vi "ShiftReg.vi"() -> ()   [LabVIEW 2012]
uses:
  <vilib>/Waveform/DTblOps.llb/DTbl Boolean Array to Digital.vi
panel:
  in  "D":bool
  out "Digital Waveform Graph":digitaldata(graph)
  in  "millisecond multiple":u32
  out "Q4":bool
  out "Q3":bool
  out "Clk":bool
  out "Q2":bool
  in  "Slices":u32
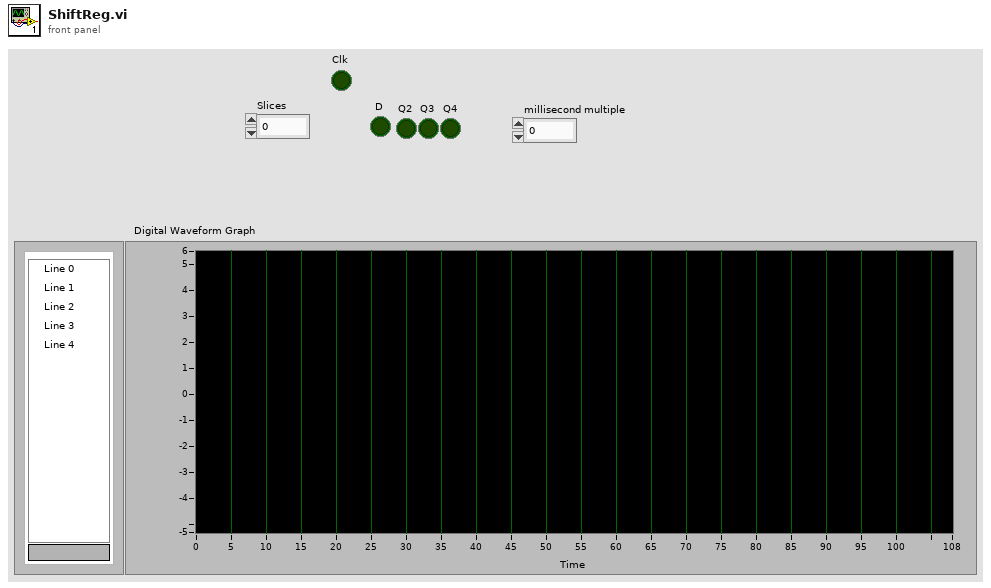
[diagram p1: front panel]
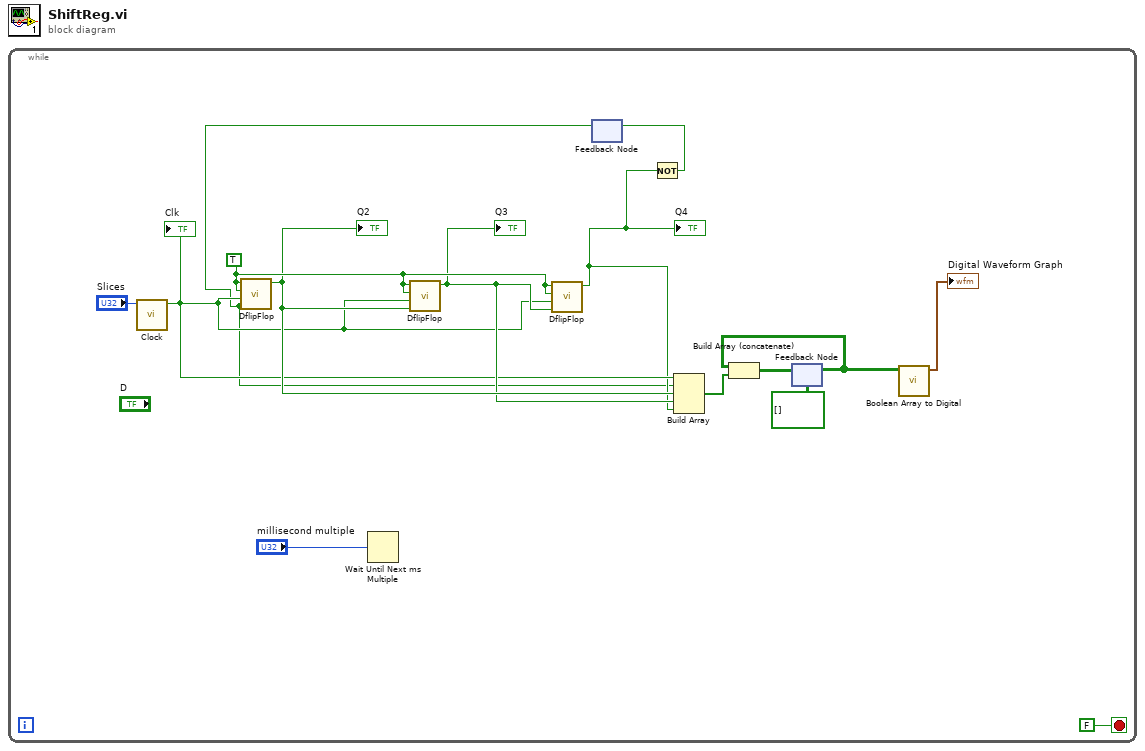
[diagram p0: block diagram]
diagram:
  n1 = while {
    stop <- FALSE stop-if-true
    w14 = TRUE ("Set")
    n2 = call "Clock.vi"("Slices"="Slices") -> ("Clk"=w4:bool)  [unwired: 10 in]
    "Clk" <- w4
    n3 = Wait Until Next ms Multiple(millisecond multiple="millisecond multiple") -> ()  [unwired: 1 out]
    n4 = feedback #1() -> (w1:bool)  [unwired: 1 in]
    n5 = call "DflipFlop.vi"("D"=w1, "Clock"=w4, "Reset"=w14, "Set"=w14) -> ("Q"=w6:bool)  [unwired: 6 in, 1 out]
    "Q2" <- w6
    n6 = call "DflipFlop.vi"("D"=w6, "Clock"=w4, "Reset"=w14, "Set"=w14) -> ("Q"=w5:bool)  [unwired: 6 in, 1 out]
    "Q3" <- w5
    n7 = call "DflipFlop.vi"("D"=w5, "Clock"=w4, "Reset"=w14, "Set"=w14) -> ("Q"=w3:bool)  [unwired: 6 in, 1 out]
    "Q4" <- w3
    n8 = Not(x=w3) -> (.not. x?=w2:bool)
    n9 = feedback-in #1(w2) -> ()
    n10 = Build Array(w4, w1, w6, w5, w3) -> (w8:bool[])
    n11 = feedback #2(bool[][] []) -> (w9:bool[][])
    n12 = Build Array (concatenate)(w9, w8) -> (w11:bool[][])
    n13 = feedback-in #2(w11) -> ()
    n14 = call-poly <vilib>:"Boolean Array to Digital.vi"("boolean array"=w9) -> ("digital data"=→"Digital Waveform Graph":digitaldata)  [unwired: 9 in, 1 out]
  }
